vi "TM624.vi"() -> ()   [LabVIEW 2019]
uses:
  <vilib>/Utility/error.llb/DialogType.ctl
  <vilib>/Platform/TimedLoop/XDataNode/timing_clust.ctl
  <vilib>/Platform/TimedLoop/XDataNode/nitl_modes.ctl
  <vilib>/Platform/TimedLoop/XDataNode/wakeup.ctl
  <vilib>/Platform/TimedLoop/XDataNode/XDataNode.xnode
  <vilib>/Platform/TimedLoop/XDataNode/XDNodeRunTimeDep.lvlib
panel:
  out "Data String":string="8/26/2022 9:42:07 AM,,,,,,,,,,,.......,.......,.......,.......,0%,0%,24.755190,23.003520,23.280240,43.286620,   0%,   0%,15.017997,0.409302,1070,1070,1068,1070,1065,1069\r,"
  in  "Tab Control 2":enum32{"Setup", "Temperature Monitor", "Notes"}(tab)
  in  "Path":path=path "C:/Users/aberryhill/Desktop"
  in  "Identifier\n(Number only e.g. 12345)":string="11885"
  in  "Description\n(cooldown)":string="cooldown"
  in  "Rate (sec)":sgl=30.0 min=1 step=5
  in  "Data Log On":bool
  in  "Go":bool
  in  "EXIT":bool
  out "Heartbeat":bool
  in  "TM6XX 1":refnum<visa-resource-name>="TCPIP0::192.168.1.5::4266::SOCKET"
  out "Chan D":string
  out "Chan C":string
  out "Chan B":string
  out "Chan A":string
  out "Temp Chart":dbl[][](graph)
  in  "Add Note":bool
  in  "Notes":string
  # "CRYOMAGNETICS, INC."
  # "General Data Logging"
  # "1)  Select Instrument I/O communication from the dropdown above.\n2)  Select the location of the data logging file, identifier, and description.\n3)  Press the Go button, the LED indicator should blink on and off every second.\n4)  When ready turn the dataloggin on by pressing the DATA LOG ON button."
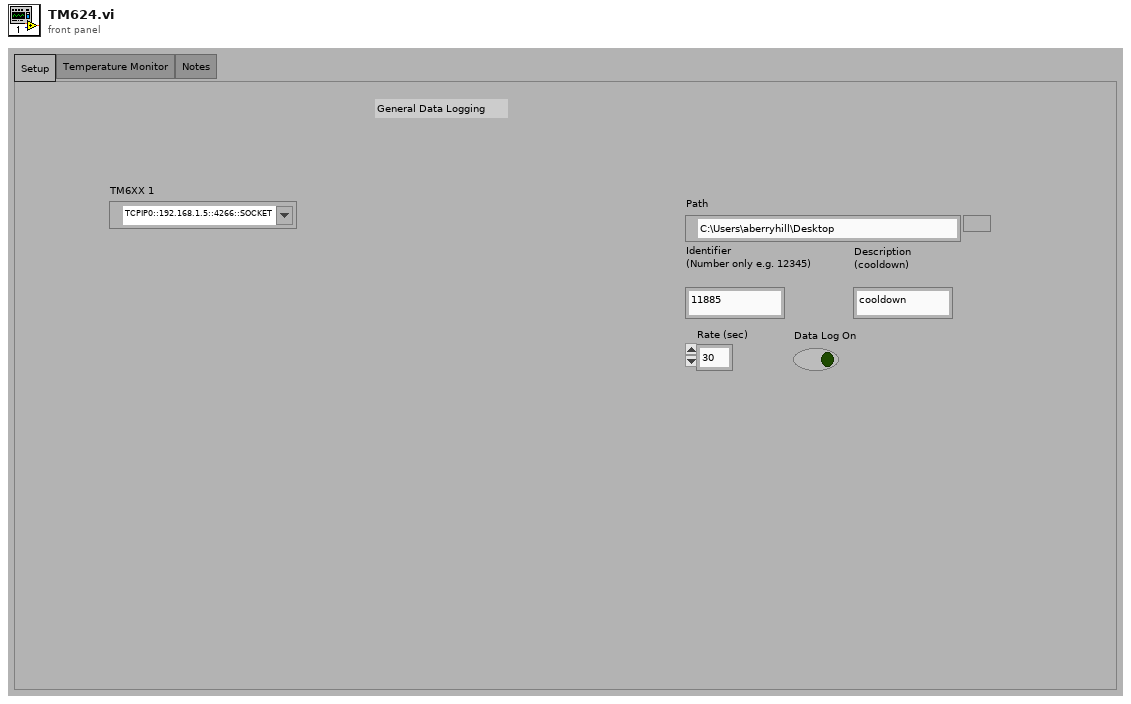
[diagram p1: front panel]
types:
  T1 = typedef "XDNodeRunTimeDep.lvlib/timing_clust.ctl" = cluster{"Expected End [f-1]":u64, "Actual End [f-1]":u64, "Finished Late? [f-1]":bool, "Expected End [i-1]":u64, "Actual End [i-1]":u64, "Finished Late? [i-1]":bool, "Expected Start [i]":u64, "Actual Start [i]":u64, "Expected Start [f]":u64, "Actual Start [f]":u64, "Source Name":string, "Structure Name":string, "Period":i64, "Deadline":i64, "Offset":i64, "Start":i64, "Priority":i32, "Timeout":i32, "Mode":T2, "Wakeup Reason":T3, "Error":errorcluster, "Source Type":string, "Secondary Source Type":string, "Global End Time":u64, "Global Start Time":u64, "Frame Duration":u64, "Iteration Duration":u64, "Assigned CPU":i32, "I/O Scan Engine Mode":u32}
  T2 = typedef "XDNodeRunTimeDep.lvlib/nitl_modes.ctl" = enum32{"No Change", "Process missed periods, maintain original phase", "Discard missed periods, maintain original phase", "Process missed periods, ignore original phase", "Discard missed periods, ignore original phase"}
  T3 = typedef "XDNodeRunTimeDep.lvlib/wakeup.ctl" = enum32{"Normal", "Aborted", "Asynchronous wakeup", "Timing source error", "Timed loop error", "Timeout"}
  T4 = enum16{"open", "replace", "create", "open or create", "replace or create", "replace or create with confirmation"}
  T5 = typedef "DialogType.ctl" = u16
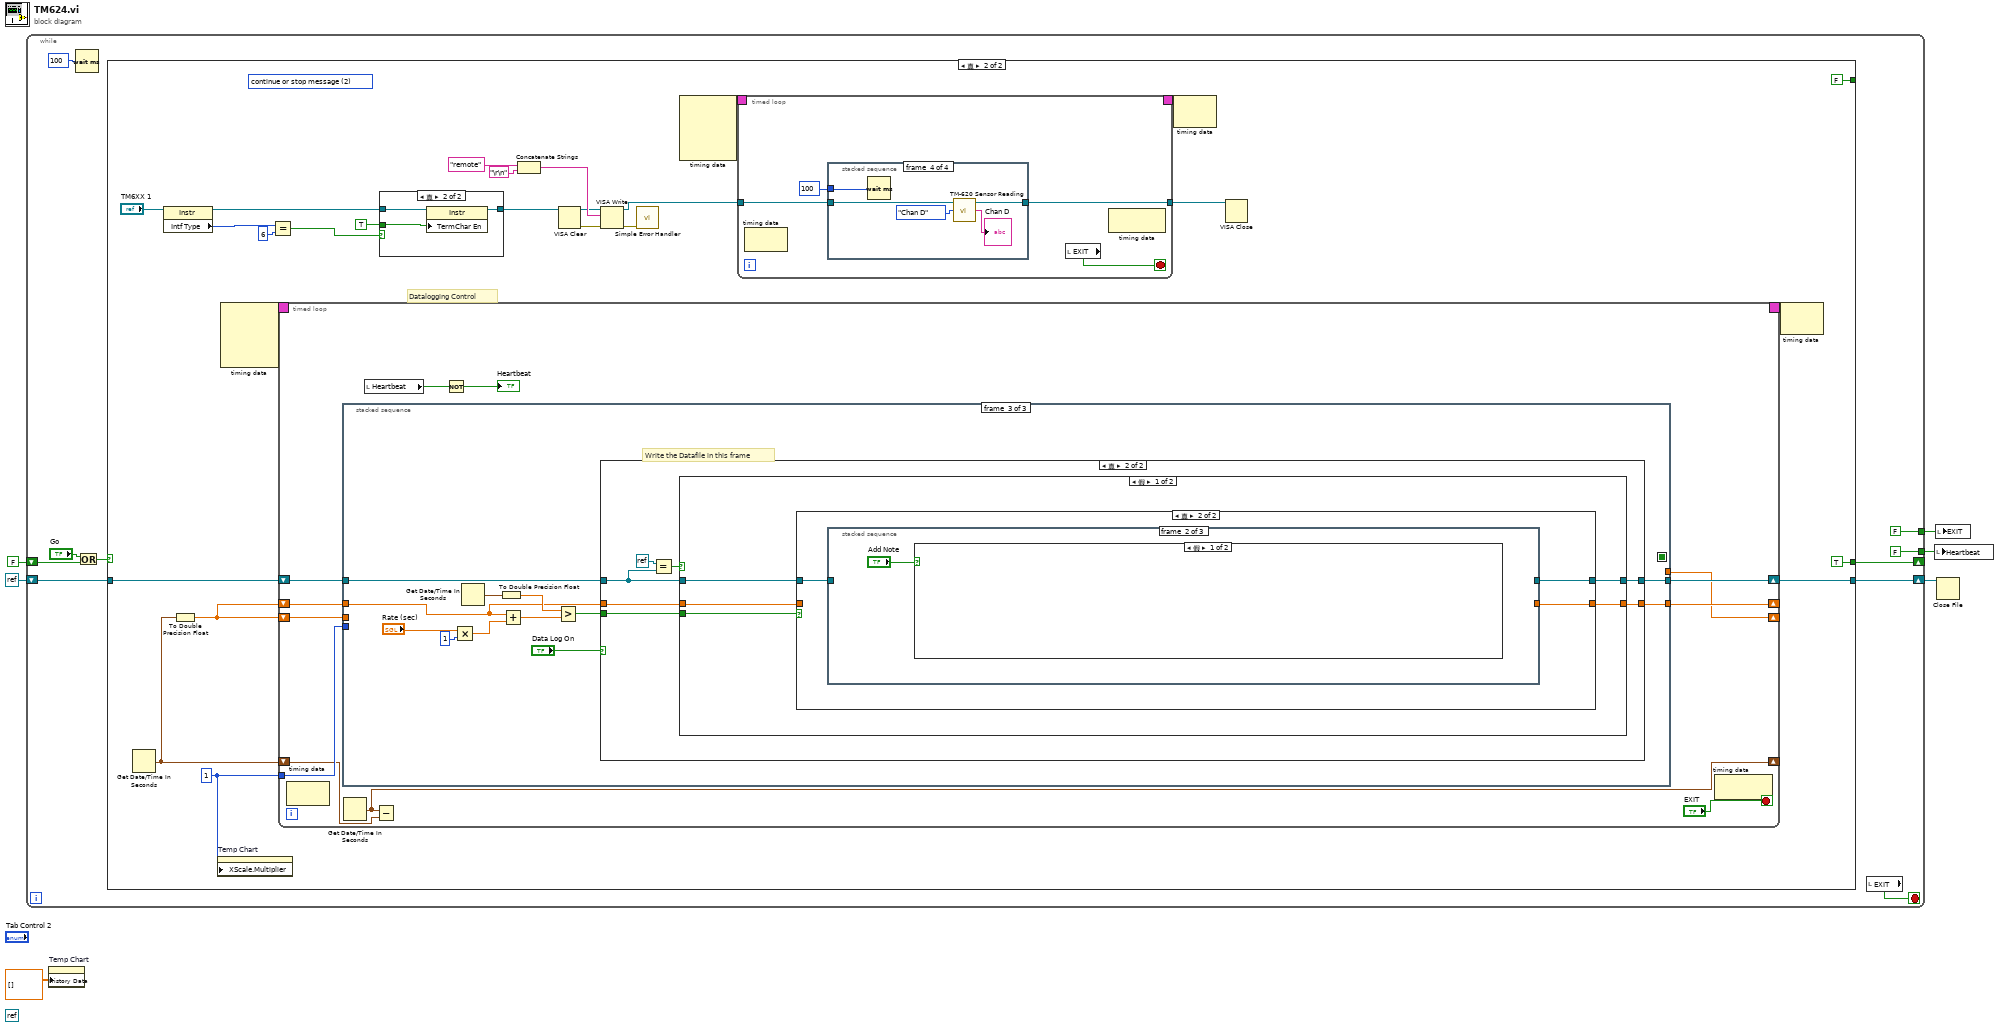
[diagram p0: block diagram]
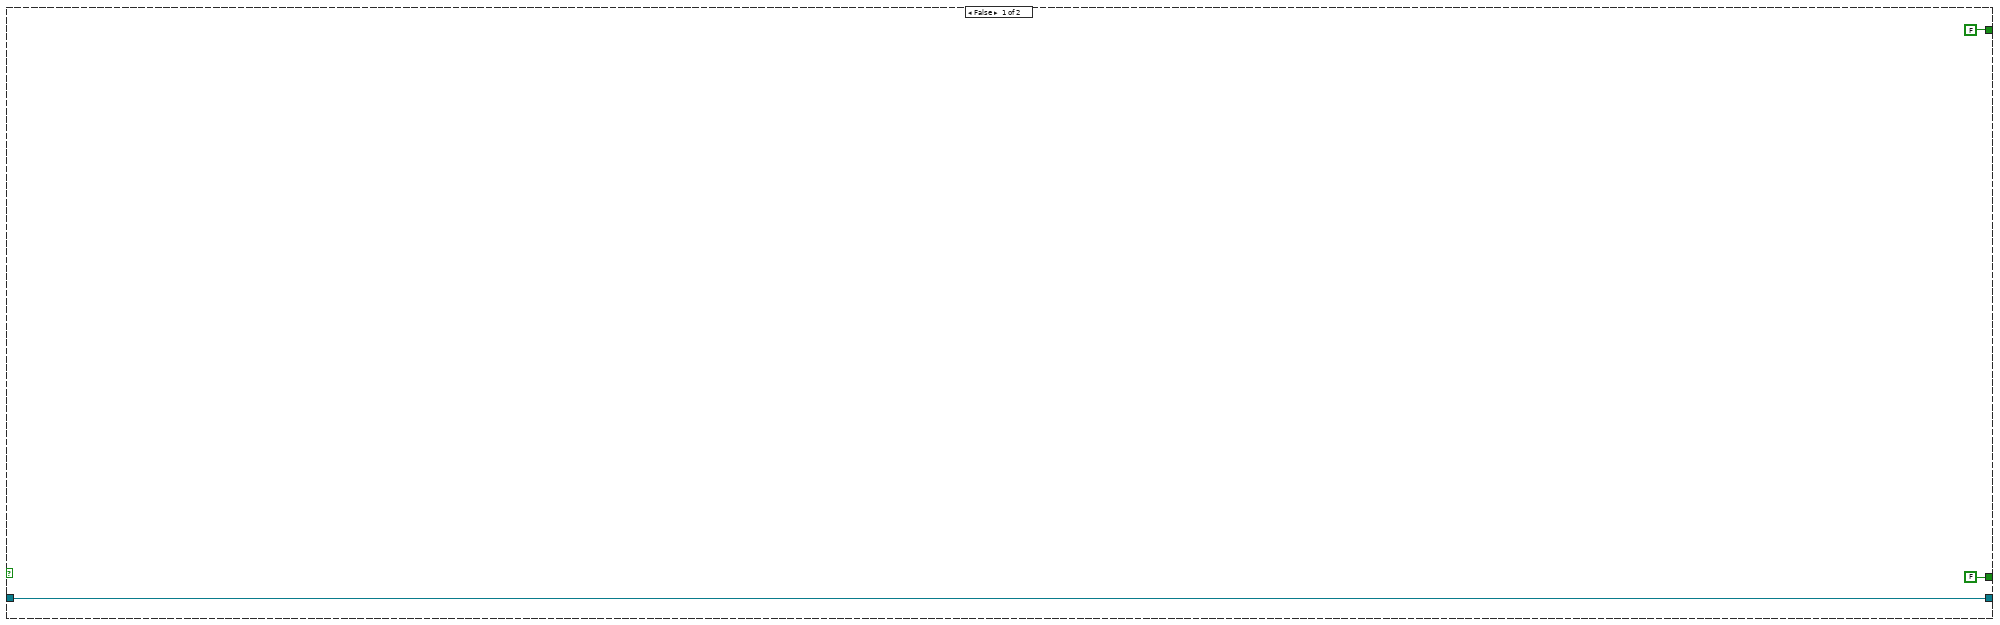
[diagram p2: hidden frame]
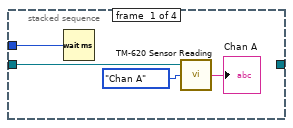
[diagram p3: hidden frame]
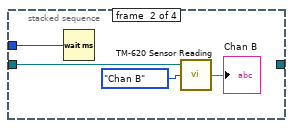
[diagram p4: hidden frame]
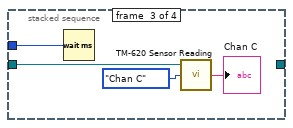
[diagram p5: hidden frame]
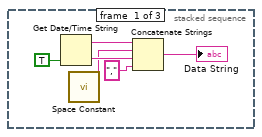
[diagram p7: hidden frame]
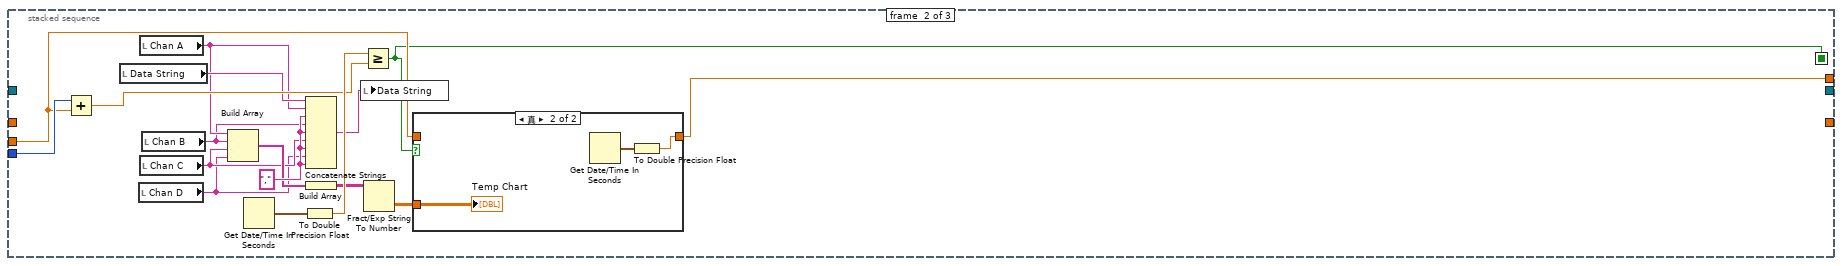
[diagram p8: hidden frame]
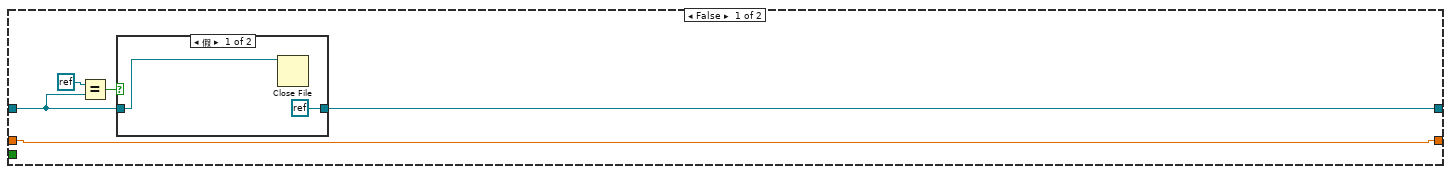
[diagram p10: hidden frame]
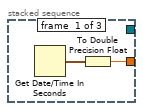
[diagram p13: hidden frame]
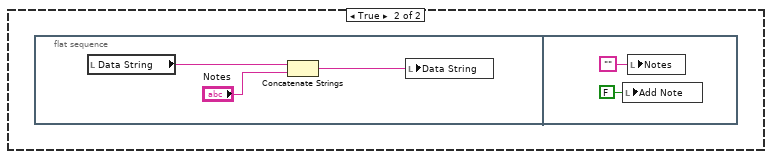
[diagram p14: hidden frame]
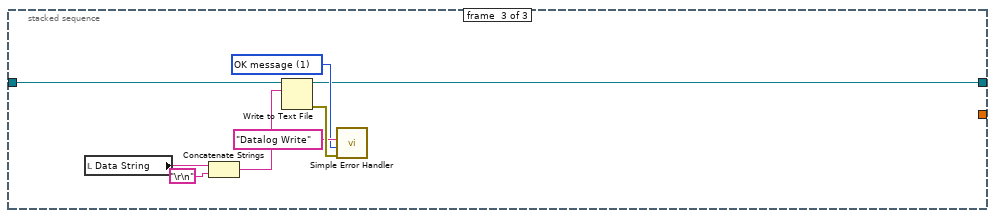
[diagram p15: hidden frame]
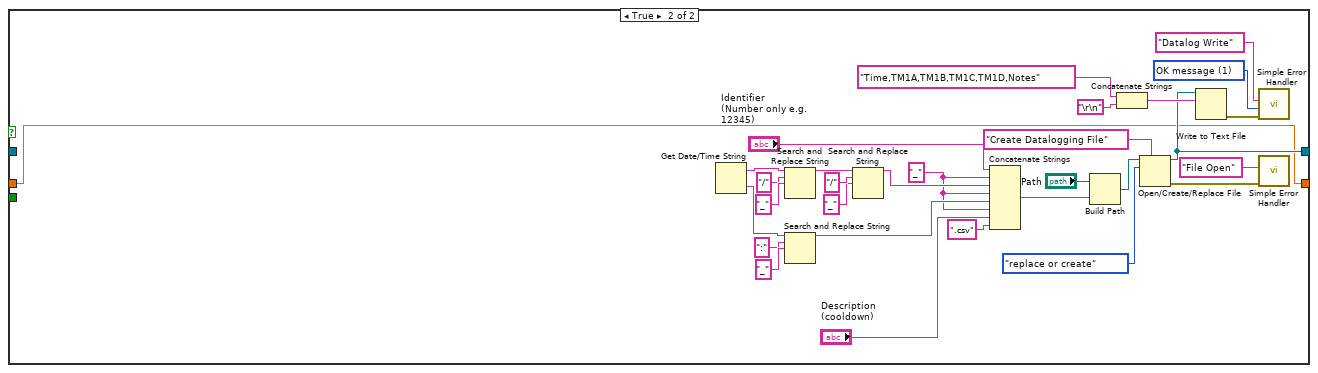
[diagram p16: hidden frame]
diagram:
  (unwired) refnum<k0> refnum
  n1 = while {
    shift-right: [w12] -> _
    shift-left: FALSE -> [w13]
    tunnel: [FALSE] -> w5
    shift-right: [w8] -> w3
    shift-left: refnum<k0> refnum -> [w9]
    tunnel: [FALSE] -> w2
    stop <- w11 stop-if-true
    n2 = Wait (ms)(milliseconds to wait=100) -> ()  [unwired: 1 out]
    n3 = Or(x="Go", y=w13) -> (x .or. y?=w14:bool)
    n4 = case shown="真" w14 {
      tunnel: [FALSE FALSE] -> _
      tunnel: [FALSE TRUE] -> w12
      tunnel: w9 -> [w17 w40]
      tunnel: [w17 w39] -> w8
      frame False {
      }
      frame True {
        (unwired) T5 2 items=["no dialog", "OK message", "continue or stop message", "OK message + warnings", "continue/stop + warnings"] ("type of dialog (OK msg:1)")
        w20 = i64 1 ("y")
        # "Datalogging Control"
        n5 = Get Date/Time In Seconds() -> (seconds since 1Jan1904=w43:timestamp)
        n6 = property class="Instr"(reference="TM6XX 1") -> (reference out=w32:refnum<visa-resource-name>, "Intf Type"=w34:u16)  [unwired: 1 in, 1 out]
        n7 = To Double Precision Float(number=w43) -> (double precision float=w31:dbl)
        n8 = property on="Temp Chart" class="WFChart (严格)"("XScale.Multiplier"=w20) -> ()  [unwired: 2 in, 2 out]
        n9 = node-c288() -> (w45:T1)  [unwired: 4 in]
        n10 = Equal?(x=w34, y=6) -> (x = y?=w35:bool)
        n11 = timed-loop {
          tunnel: w20 -> [w86]
          timing: w45 -> [_]
          timing-out: [_] -> w44
          shift-right: [w84] -> w39
          shift-left: w40 -> [w85]
          shift-right: [w82] -> _
          shift-left: w43 -> [w83]
          shift-right: [w78] -> _
          shift-left: w31 -> [w79]
          shift-right: [w76] -> _
          shift-left: w31 -> [w77]
          stop <- "EXIT" stop-if-true
          n12 = node-c288() -> ()  [unwired: 1 in, 1 out]
          n13 = stacked-sequence {
            seq-local: [_ w102 _] -> [_ _ _]
            tunnel: w86 -> [_ w108 _]
            tunnel: w85 -> [_ _ w125]
            tunnel: [_ _ w126] -> w84
            tunnel: w79 -> [_ _ w116]
            tunnel: [_ _ w117] -> w78
            tunnel: w77 -> [_ w106 _]
            tunnel: [_ w107 _] -> w76
            frame #0 {
              n14 = Get Date/Time String(want seconds? (F)=TRUE) -> (date string=w93:string, time string=w91:string)  [unwired: 2 in]
              n15 = call <vilib>:"Space Constant.vi"() -> ("String"=w90:string)
              n16 = Concatenate Strings(w93, w90, w91, "," ("element")) -> (→"Data String":string)
            }
            frame #1 {
              w101 = ","
              n17 = Add(x=w108, y=w106) -> (x+y=w110:dbl)
              n18 = local read "Data String"() -> (w104:string)
              n19 = local read "Chan D"() -> (w95:string)
              n20 = local read "Chan A"() -> (w98:string)
              n21 = local read "Chan C"() -> (w96:string)
              n22 = local read "Chan B"() -> (w97:string)
              n23 = Build Array(w98, w97, w96, w95) -> (w100:string[])
              n24 = Get Date/Time In Seconds() -> (seconds since 1Jan1904=w109:timestamp)
              n25 = To Double Precision Float(number=w109) -> (double precision float=w111:dbl)
              n26 = Concatenate Strings(w104, w98, w101, w97, w101, w96, w101, w95, w101) -> (w103:string)
              n27 = Build Array(w100) -> (w99:string[][])
              n28 = local write "Data String"(w103) -> ()
              n29 = Greater Or Equal?(x=w111, y=w110) -> (x >= y?=w102:bool)
              n30 = Fract/Exp String To Number(string=w99) -> (number=w105:dbl[][])  [unwired: 3 in, 1 out]
              n31 = case shown="真" w102 {
                tunnel: w105 -> [_ w114]
                tunnel: [w112 w113] -> w107
                tunnel: w106 -> [w112 _]
                frame False {
                }
                frame True {
                  n32 = Get Date/Time In Seconds() -> (seconds since 1Jan1904=w115:timestamp)
                  n33 = To Double Precision Float(number=w115) -> (double precision float=w113:dbl)
                  "Temp Chart" <- w114
                }
              }
            }
            frame #2 {
              # "Write the Datafile in this frame"
              n34 = Multiply(x="Rate (sec)", y=i16 1) -> (x*y=w119:sgl)
              n35 = Get Date/Time In Seconds() -> (seconds since 1Jan1904=w122:timestamp)
              n36 = To Double Precision Float(number=w122) -> (double precision float=w124:dbl)
              n37 = Add(x=w116, y=w119) -> (x+y=w123:dbl)
              n38 = Greater?(x=w124, y=w123) -> (0:w121:bool)
              n39 = case shown="真" "Data Log On" {
                tunnel: w125 -> [w132 w141]
                tunnel: [w131 w140] -> w126
                tunnel: w121 -> [_ w138]
                tunnel: [w128 w137] -> w117
                tunnel: w116 -> [w128 w136]
                frame False {
                  n40 = Equal?(x=refnum<k0> refnum, y=w132) -> (x = y?=w129:bool)
                  n41 = case shown="假" w129 {
                    tunnel: w132 -> [w134 w135]
                    tunnel: [refnum<k0> refnum w135] -> w131
                    frame False {
                      n42 = Close File(refnum=w134) -> ()  [unwired: 1 in, 2 out]
                    }
                    frame True {
                    }
                  }
                }
                frame True {
                  n43 = Equal?(x=refnum<k0> refnum, y=w141) -> (x = y?=w142:bool)
                  n44 = case shown="假" w142 {
                    tunnel: w141 -> [w147 _]
                    tunnel: [w146 w191] -> w140
                    tunnel: w138 -> [w145 _]
                    tunnel: [w144 w172] -> w137
                    tunnel: w136 -> [w143 w172]
                    frame False {
                      n45 = case shown="真" w145 {
                        tunnel: w147 -> [w149 w152]
                        tunnel: [w149 w151] -> w146
                        tunnel: [w148 w150] -> w144
                        tunnel: w143 -> [w148 _]
                        frame False {
                        }
                        frame True {
                          n46 = stacked-sequence {
                            tunnel: w152 -> [_ _ w163]
                            tunnel: [_ _ w162] -> w151
                            tunnel: [w153 _ _] -> w150
                            frame #0 {
                              n47 = Get Date/Time In Seconds() -> (seconds since 1Jan1904=w154:timestamp)
                              n48 = To Double Precision Float(number=w154) -> (double precision float=w153:dbl)
                            }
                            frame #1 {
                              n49 = case shown="假" "Add Note" {
                                frame False {
                                }
                                frame True {
                                n50 = flat-sequence {
                                frame #0 {
                                n51 = local read "Data String"() -> (w156:string)
                                n52 = Concatenate Strings(w156, "Notes") -> (w157:string)
                                n53 = local write "Data String"(w157) -> ()
                                }
                                frame #1 {
                                n54 = local write "Add Note"(FALSE ("Add Note")) -> ()
                                n55 = local write "Notes"("" ("Notes")) -> ()
                                }
                                }
                                }
                              }
                            }
                            frame #2 {
                              w166 = u16 1 items=["no dialog", "OK message", "continue or stop message"] ("type of dialog (OK msg:1)")
                              n56 = local read "Data String"() -> (w161:string)
                              n57 = Concatenate Strings(w161, "\r\n") -> (w164:string)
                              n58 = Write to Text File(file (use dialog)=w163, text=w164) -> (refnum out=w162:refnum<file>, error out=w168:errorcluster)  [unwired: 2 in, 1 out]
                              n59 = call "Simple Error Handler.vi"("error source (\" \")"="Datalog Write" ("error source (\" \")"), "type of dialog (OK msg:1)"=w166, "error in (no error)"=w168) -> ()  [unwired: 2 in, 5 out]
                            }
                          }
                        }
                      }
                    }
                    frame True {
                      w177 = "_"
                      w194 = u16 1 items=["no dialog", "OK message", "continue or stop message"] ("type of dialog (OK msg:1)")
                      n60 = Get Date/Time String() -> (date string=w183:string, time string=w185:string)  [unwired: 3 in]
                      n61 = Search and Replace String(input string=w183, search string="/", replace string="_" ("replace string (\"\")")) -> (result string=w186:string)  [unwired: 5 in, 3 out]
                      n62 = Search and Replace String(input string=w185, search string=":", replace string="_" ("replace string (\"\")")) -> (result string=w178:string)  [unwired: 5 in, 3 out]
                      n63 = Search and Replace String(input string=w186, search string="/", replace string="_" ("replace string (\"\")")) -> (result string=w187:string)  [unwired: 5 in, 3 out]
                      n64 = Concatenate Strings("Identifier\n(Number only e.g. 12345)", w177, w187, w177, w178, w177, "Description\n(cooldown)", ".csv") -> (w170:string)
                      n65 = Build Path(base path="Path", name or relative path=w170) -> (appended path=w171:path)
                      n66 = Concatenate Strings("Time,TM1A,TM1B,TM1C,TM1D,Notes" ("Data String"), "\r\n") -> (w192:string)
                      n67 = Open/Create/Replace File(file path (use dialog)=w171, prompt="Create Datalogging File", operation (0:open)=T4."replace or create") -> (refnum out=w191:refnum<file>, error out=w197:errorcluster)  [unwired: 3 in, 1 out]
                      n68 = Write to Text File(file (use dialog)=w191, text=w192) -> (error out=w196:errorcluster)  [unwired: 2 in, 2 out]
                      n69 = call "Simple Error Handler.vi"("error source (\" \")"="Datalog Write" ("error source (\" \")"), "type of dialog (OK msg:1)"=w194, "error in (no error)"=w196) -> ()  [unwired: 2 in, 5 out]
                      n70 = call "Simple Error Handler.vi"("error source (\" \")"="File Open" ("error source (\" \")"), "error in (no error)"=w197) -> ()  [unwired: 3 in, 5 out]
                    }
                  }
                }
              }
            }
          }
          n71 = Get Date/Time In Seconds() -> (seconds since 1Jan1904=w82:timestamp)
          n72 = local read "Heartbeat"() -> (w81:bool)
          n73 = Subtract(x=w82, y=w83) -> ()  [unwired: 1 out]
          n74 = Not(x=w81) -> (.not. x?=→"Heartbeat":bool)
          n75 = node-c288() -> ()  [unwired: 1 in, 1 out]
        }
        n76 = case shown="真" w35 {
          tunnel: [w71 w72] -> w38
          tunnel: TRUE -> [_ w74]
          tunnel: w32 -> [w71 w73]
          frame False {
          }
          frame True {
            n77 = property class="Instr"(reference=w73, "TermChar En"=w74) -> (reference out=w72:refnum<visa-resource-name>)  [unwired: 1 in, 1 out]
          }
        }
        n78 = Concatenate Strings("remote" ("write buffer (\"\")"), "\r\n") -> (w25:string)
        n79 = VISA Clear(VISA resource name=w38) -> (VISA resource name out=w22:refnum<visa-resource-name>, error out=w21:errorcluster)  [unwired: 1 in]
        n80 = VISA Write(VISA resource name=w22, write buffer=w25, error in (no error)=w21) -> (VISA resource name out=w27:refnum<visa-resource-name>, error out=w24:errorcluster)  [unwired: 1 out]
        n81 = call "Simple Error Handler.vi"("error in (no error)"=w24) -> ()  [unwired: 4 in, 5 out]
        n82 = node-c288() -> (w30:T1)  [unwired: 4 in]
        n83 = timed-loop {
          tunnel: w27 -> [w48]
          timing: w30 -> [_]
          timing-out: [_] -> w29
          tunnel: [w47] -> w28
          stop <- w46 stop-if-true
          n84 = node-c288() -> ()  [unwired: 1 in, 1 out]
          n85 = stacked-sequence {
            tunnel: w48 -> [w53 w57 w61 w66]
            tunnel: u32 100 ("milliseconds to wait") -> [w55 w59 w63 w68]
            tunnel: [_ _ _ w65] -> w47
            frame #0 {
              n86 = Wait (ms)(milliseconds to wait=w55) -> ()  [unwired: 1 out]
              n87 = call "TM-620 Sensor Reading.vi"("channel"=enum16{"Chan A", "Chan B", "Chan C", "Chan D"}."Chan A", "VISA session"=w53) -> ("response out"=→"Chan A":string)  [unwired: 1 in, 2 out]
            }
            frame #1 {
              n88 = Wait (ms)(milliseconds to wait=w59) -> ()  [unwired: 1 out]
              n89 = call "TM-620 Sensor Reading.vi"("channel"=enum16{"Chan A", "Chan B", "Chan C", "Chan D"}."Chan B", "VISA session"=w57) -> ("response out"=→"Chan B":string)  [unwired: 1 in, 2 out]
            }
            frame #2 {
              n90 = Wait (ms)(milliseconds to wait=w63) -> ()  [unwired: 1 out]
              n91 = call "TM-620 Sensor Reading.vi"("channel"=enum16{"Chan A", "Chan B", "Chan C", "Chan D"}."Chan C", "VISA session"=w61) -> ("response out"=→"Chan C":string)  [unwired: 1 in, 2 out]
            }
            frame #3 {
              n92 = Wait (ms)(milliseconds to wait=w68) -> ()  [unwired: 1 out]
              n93 = call "TM-620 Sensor Reading.vi"("channel"=enum16{"Chan A", "Chan B", "Chan C", "Chan D"}."Chan D", "VISA session"=w66) -> ("response out"=→"Chan D":string, "dup VISA session"=w65:refnum<visa-resource-name>)  [unwired: 1 in, 1 out]
            }
          }
          n94 = local read "EXIT"() -> (w46:bool)
          n95 = node-c288() -> ()  [unwired: 1 in, 1 out]
        }
        n96 = node-c288(w29) -> ()  [unwired: 1 out]
        n97 = VISA Close(VISA resource name=w28) -> ()  [unwired: 1 in, 1 out]
        n98 = node-c288(w44) -> ()  [unwired: 1 out]
      }
    }
    n99 = local read "EXIT"() -> (w11:bool)
  }
  n100 = property on="Temp Chart" class="WFChart (严格)"("History Data"=dbl[][] []) -> ()  [unwired: 2 in, 2 out]
  n101 = local write "Heartbeat"(w2) -> ()
  n102 = local write "EXIT"(w5) -> ()
  n103 = Close File(refnum=w3) -> ()  [unwired: 1 in, 2 out]
